vi "DrawROICircle.vi"(0 "old picture":picture, 1 "ROI?":bool, 2 "Radius (G/S)":dbl, 3 "Center (G/S)":cluster{dbl, dbl}, 4 "PicSize":u32=360, 5 "Color":u32(colorbox)=16744512, 6 "G_max":dbl=1.1, 7 "S_max":dbl=1.1, 8 "G_min":dbl=-0.1, 9 "S_min":dbl=-0.1) -> (14 "new picture":picture)   [LabVIEW 2015]
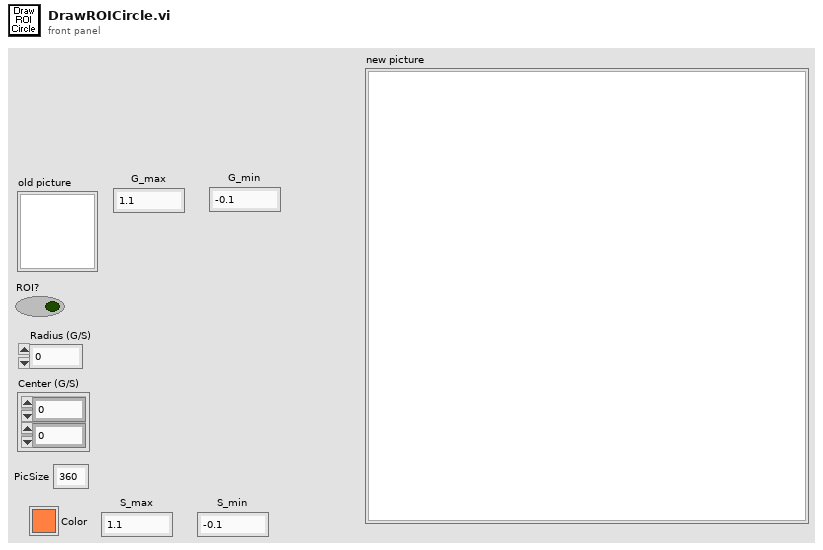
[diagram p1: front panel]
types:
  T1 = cluster{"Width":u16, "Style":enum32{"Solid", "Dash", "Dot", "DashDot", "DashDotDot"}}
  T2 = cluster{"G_min":dbl, "S_max":dbl, "G_min":dbl, "S_max":dbl}
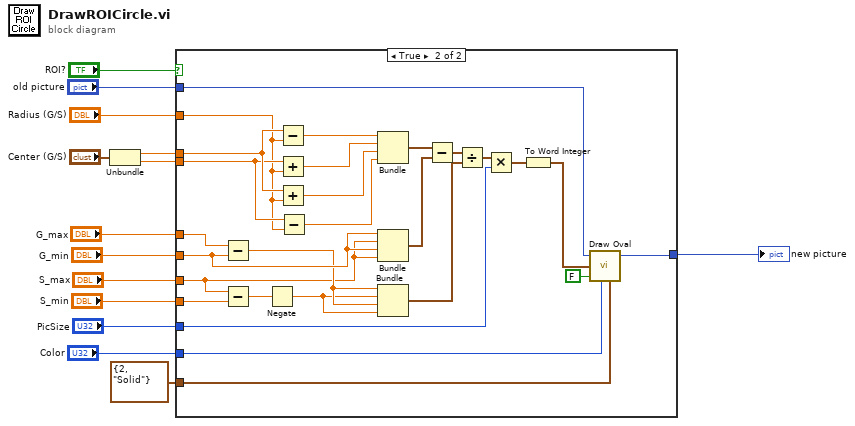
[diagram p0: block diagram]
diagram:
  n1 = Unbundle("Center (G/S)") -> (w3:dbl, w1:dbl)
  n2 = case shown="True" "ROI?" {
    tunnel: "old picture" -> [w15 w21]
    tunnel: "Radius (G/S)" -> [_ w16]
    tunnel: "Color" -> [_ w40]
    tunnel: T1 {"Width"=2, "Style"=enum."Solid"} ("pen") -> [_ w39]
    tunnel: [w15 w42] -> w13
    tunnel: "G_max" -> [_ w38]
    tunnel: "G_min" -> [_ w31]
    tunnel: "S_max" -> [_ w19]
    tunnel: "S_min" -> [_ w30]
    tunnel: "PicSize" -> [_ w23]
    tunnel: w3 -> [_ w37]
    tunnel: w1 -> [_ w20]
    frame False {
    }
    frame True {
      n3 = Subtract(x=w38, y=w31) -> (x-y=w27:dbl)
      n4 = Subtract(x=w19, y=w30) -> (x-y=w18:dbl)
      n5 = Negate(x=w18) -> (-x=w17:dbl)
      n6 = Subtract(x=w37, y=w16) -> (x-y=w36:dbl)
      n7 = Add(x=w20, y=w16) -> (x+y=w35:dbl)
      n8 = Add(x=w37, y=w16) -> (x+y=w34:dbl)
      n9 = Subtract(x=w20, y=w16) -> (x-y=w33:dbl)
      n10 = Bundle(w36, w35, w34, w33) -> (w29:cluster{dbl, dbl, dbl, dbl})  [unwired: 1 in]
      n11 = Bundle("G_min"=w31, "S_max"=w19, "G_min"=w31, "S_max"=w19) -> (w28:T2)  [unwired: 1 in]
      n12 = Bundle(w27, w17, w27, w17) -> (w25:cluster{dbl, dbl, dbl, dbl})  [unwired: 1 in]
      n13 = Subtract(x=w29, y=w28) -> (x-y=w26:cluster{dbl, dbl, dbl, dbl})
      n14 = Divide(x=w26, y=w25) -> (x/y=w24:cluster{dbl, dbl, dbl, dbl})
      n15 = Multiply(x=w24, y=w23) -> (x*y=w22:cluster{dbl, dbl, dbl, dbl})
      n16 = To Word Integer(number=w22) -> (16bit integer=w32:cluster{i16, i16, i16, i16})
      n17 = call <vilib>:"Draw Oval.vi"("picture"=w21, "rect"=w32, "fill?(F)"=FALSE, "color(black)"=w40, "pen"=w39) -> ("new picture"=w42:picture)  [unwired: 4 in]
    }
  }
  "new picture" <- w13
